vi "GOOP_MyComputer_Item_OnPopUpMenu.vi"(11 "Object":u64) -> ()   [LabVIEW 2012]
uses:
  <resource>/Framework/Providers/API/mxLvMenuItem.ctl
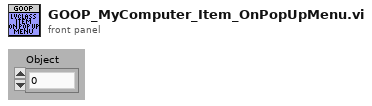
[diagram p1: front panel]
types:
  T1 = typedef "mxLvMenuItem.ctl" = cluster{"Menu Name":string, "Description":string, "Icon File Name":path, "Menu Tag":string, "Enabled":bool, "Checked":bool, "Separator":bool, "Batchable":bool, "Weight":i32, "Batch Mode (Ignored if Not Batchable)":enum32{"Show If All Items Support Command", "Show If Any Items Support Command"}, "Menu Location":enum32{"<None>", "Project", "Project / Build Specifications", "Tools", "Tools / Source Control", "Tools / Real-Time Module", "Help"}, "Exclude From Getting Started Window Menu":bool}
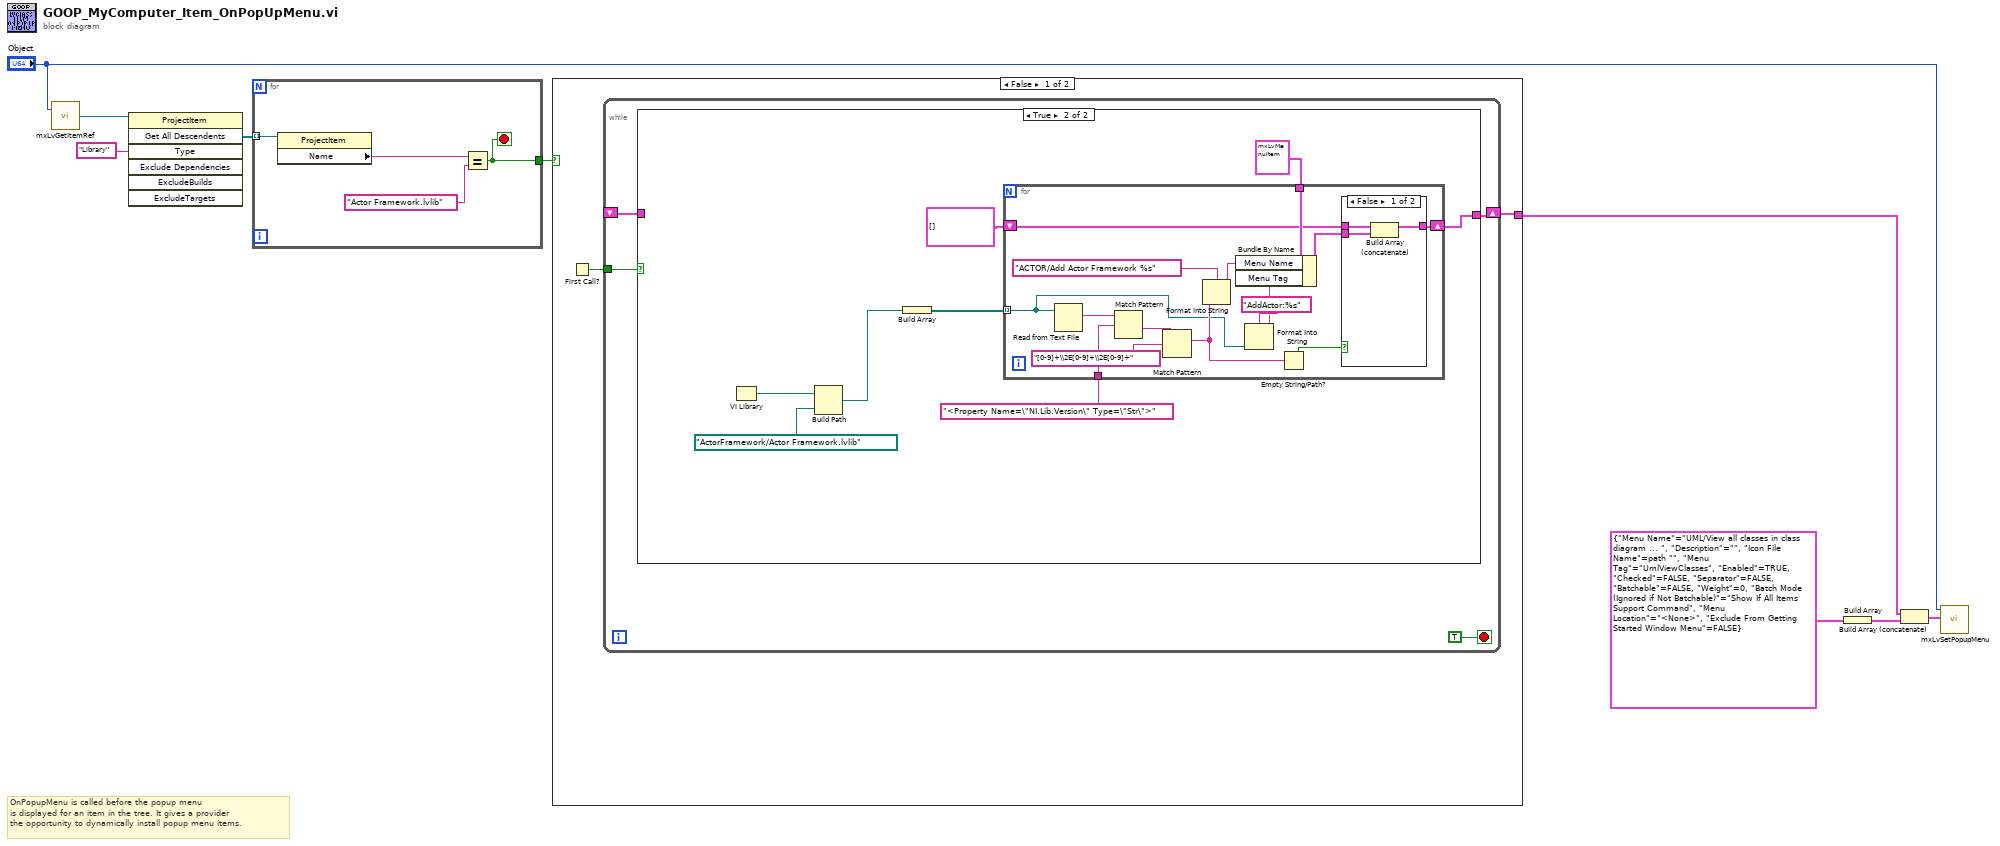
[diagram p0: block diagram]
diagram:
  # "OnPopupMenu is called before the popup menu\nis displayed for an item in the tree. It gives a provider\nthe opportunity to dynamically install popup menu items."
  n1 = call <resource>:"mxLvGetItemRef.vi"("Item"="Object") -> ("Item Refnum"=w5:refnum<vi>)  [unwired: 1 in, 2 out]
  n2 = invoke class="ProjectItem" method="Get All Descendents"(reference=w5, "Type"="Library") -> ("All Descendents"=w3:refnum<vi>[])  [unwired: 5 in, 6 out]
  n3 = for {
    tunnel: w3 -> [w13] mode=indexing
    tunnel: [w11] -> w2
    stop <- w11 stop-if-true
    n4 = property class="ProjectItem"(reference=w13) -> ("Name"=w10:string)  [unwired: 1 in, 2 out]
    n5 = Equal?(x=w10, y="Actor Framework.lvlib") -> (x = y?=w11:bool)
  }
  n6 = case shown="False" w2 {
    tunnel: [w15 _] -> w7
    frame False {
      n7 = First Call?() -> (First Call?: T/F=w14:bool)
      n8 = while {
        shift-right: [w19] -> w15
        shift-left: _ -> [w16]
        tunnel: w14 -> [w17]
        stop <- TRUE stop-if-true
        n9 = case shown="True" w17 {
          tunnel: [w20 w21] -> w19
          tunnel: w16 -> [w20 _]
          frame False {
          }
          frame True {
            n10 = VI Library() -> (path=w27:path)
            n11 = Build Path(base path=w27, name or relative path=path "ActorFramework/Actor Framework.lvlib" ("stripped path")) -> (appended path=w25:path)
            n12 = Build Array(w25) -> (w28:path[])
            n13 = for {
              tunnel: w28 -> [w29] mode=indexing
              tunnel: "<Property Name=\"NI.Lib.Version\" Type=\"Str\">" ("regular expression") -> [w42]
              tunnel: T1 {"Menu Name"="ACTOR/Add Actor Framework", "Description"="", "Icon File Name"=path "", "Menu Tag"="AddActor", "Enabled"=TRUE, "Checked"=FALSE, "Separator"=FALSE, "Batchable"=FALSE, "Weight"=0, "Batch Mode (Ignored if Not Batchable)"=enum."Show If All Items Support Command", "Menu Location"=enum."<None>", "Exclude From Getting Started Window Menu"=FALSE} ("Menu Item") -> [w39]
              shift-right: [w30] -> w21
              shift-left: T1[] [] -> [w32]
              n14 = Read from Text File(file (use dialog)=w29) -> (text=w43:string)  [unwired: 3 in, 3 out]
              n15 = Match Pattern(string=w43, regular expression=w42) -> (after substring=w41:string)  [unwired: 1 in, 3 out]
              n16 = Match Pattern(string=w41, regular expression="[0-9]+\\2E[0-9]+\\2E[0-9]+") -> (match substring=w34:string)  [unwired: 1 in, 3 out]
              n17 = Format Into String(format string="ACTOR/Add Actor Framework %s" ("Menu Name"), w34) -> (resulting string=w37:string)  [unwired: 2 in, 1 out]
              n18 = Format Into String(format string="AddActor:%s" ("Menu Tag"), w29) -> (resulting string=w35:string)  [unwired: 2 in, 1 out]
              n19 = Bundle By Name(cluster=w39, "Menu Name"=w37, "Menu Tag"=w35) -> (w31:T1)
              n20 = Empty String/Path?(string/path=w34) -> (empty?=w33:bool)
              n21 = case shown="False" w33 {
                tunnel: w32 -> [w46 w47]
                tunnel: w31 -> [w45 _]
                tunnel: [w44 w47] -> w30
                frame False {
                  n22 = Build Array (concatenate)(w46, w45) -> (w44:T1[])
                }
                frame True {
                }
              }
            }
          }
        }
      }
    }
    frame True {
    }
  }
  n23 = Build Array(T1 {"Menu Name"="UML/View all classes in class diagram ... ", "Description"="", "Icon File Name"=path "", "Menu Tag"="UmlViewClasses", "Enabled"=TRUE, "Checked"=FALSE, "Separator"=FALSE, "Batchable"=FALSE, "Weight"=0, "Batch Mode (Ignored if Not Batchable)"=enum."Show If All Items Support Command", "Menu Location"=enum."<None>", "Exclude From Getting Started Window Menu"=FALSE} ("Menu Item")) -> (w9:T1[])
  n24 = Build Array (concatenate)(w7, w9) -> (w8:T1[])
  n25 = call <resource>:"mxLvSetPopupMenu.vi"("Popup Menu Items"=w8, "Item"="Object") -> ()  [unwired: 8 in, 2 out]
